vi "Controller.vi"(8 "error in":errorcluster) -> ()   [LabVIEW 2016, in "Vision Drive.lvlib"]
uses:
  Vision Drive.lvlib
  Target to Robot.ctl
  <vilib>/Analysis/coordinate.llb/Euler Rotation Order.ctl
  Constants/Private/Private Global.vi
  Private/Vision Target Global.vi
  Vision Server/Vision Server.lvclass
  Constants/Constants.lvlib
  <vilib>/Analysis/NI_AALPro.lvlib
  <vilib>/Analysis/coordinate.llb/3D Cartesian Coordinate Rotation (Euler) (Scalar).vi
panel:
  out "Pitch":dbl
  out "timestamp":u32
  out "Target Found?":bool
  out "Distance":dbl
  out "Angle":dbl
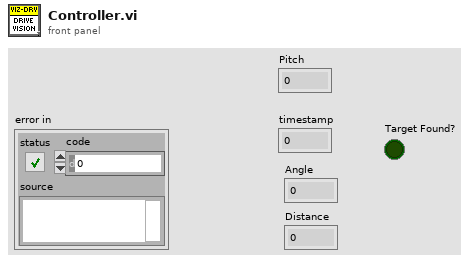
[diagram p1: front panel]
types:
  T1 = typedef "Constants.lvlib/Constants.ctl" = cluster{"Port Layout":cluster{"RightMotorInverted":bool, "LeftMotorInverted":bool, "Left Motors":T2, "Right Motors":T2, "Auton List":string[], "XBOX Port":T3, "Encoder L A":T4, "Encoder L B":T4, "Encoder R A":T4, "Encoder R B":T4, "L Encoder Inverse":bool, "R Encoder Inverse":bool, "Drive Distance per Count":dbl, "Gyro Bus":T5, "Fuel Roller 1":T2, "Front Roller":T2, "Gear Flipper":T2, "Climber 1":T2, "Fuel Roller Invert":bool, "Front Roller Invert":bool, "Gear Flipper Invert":bool, "Climber Invert":bool, "PCM":u8, "Fuel Roller 2":T2, "Gear Sensor":T6, "Gear Release Fwd":T7, "Gear Release Rvrs":T7, "Fuel Arm Fwd":T7, "Fuel Arm Rvrs":T7, "Shifter Fwrd":T7, "Shifter Rvrs":T7, "Climber 2":T2, "PDP":u8, "Shooter Front Channel":u8, "Shooter Rear Channel":u8, "Shooter Feed Channel":u8, "Camera Servo":T2, "Gear Servo":T2, "Gear Puncher Fwrd":T7, "Gear Puncher Rvrs":T7, "Shooter Inverse":bool, "Ring Light Switch":T4}, "Drive Constants":cluster{"Wheelbase In.":dbl, "Max Velocity (In/sec)":dbl, "Max Accel (In/sec^2)":dbl, "Max Jerk (In/sec^3)":dbl, "Path dt":dbl, "Path Sample Count":i32, "Deadband":dbl}, "Arm System":cluster{"Front Roller Gear Speed":dbl, "Front Roller Fuel Speed":dbl, "Gear Flipper Speed":dbl, "Fuel Roller Speed":dbl, "Gear Release Wait (ms)":i32, "Gear Sensor Threshold":dbl, "Flappy Open Angle":i32, "Flappy Close Angle":i32, "Ramp Rate (EGU/min)":dbl}, "Shooter":cluster{"Shooter Wheels":cluster{"P":dbl, "I":dbl, "D":dbl, "F":dbl, "IZone":dbl}, "Feeder":cluster{"P":dbl, "I":dbl, "D":dbl, "F":dbl, "IZone":dbl}, "Front Shooter RPM":dbl, "Rear Shooter RPM":dbl, "Agitator Speed":dbl, "Feeder Speed":dbl, "Shooter CPR":u32, "Feeder CPR":u32}, "Vision":cluster{"High Goal Height (in.)":dbl, "Low Goal Height (in.)":dbl, "Camera Height High (in.)":dbl, "Camera Height Low (in.)":dbl, "Servo Pitch Gear (deg)":dbl, "Camera Yaw (deg)":dbl, "Servo Gear":i32, "Servo Boiler":i32, "Servo Pitch Boiler (deg)":dbl}}
  T2 = typedef "FPGA_DIOPWMChannel.ctl" = enum8{"PWM 0", "PWM 1", "PWM 2", "PWM 3", "PWM 4", "PWM 5", "PWM 6", "PWM 7", "PWM 8", "PWM 9", "PWM MXP 0", "PWM MXP 1", "PWM MXP 2", "PWM MXP 3", "PWM MXP 4", "PWM MXP 5", "PWM MXP 6", "PWM MXP 7", "PWM MXP 8", "PWM MXP 9", "Invalid"}
  T3 = typedef "WPI_JoystickDeviceEnum.ctl" = enum16{"USB 0", "USB 1", "USB 2", "USB 3", "USB 4", "USB 5"}
  T4 = typedef "FPGA_DIOChannel.ctl" = enum8{"DIO 0", "DIO 1", "DIO 2", "DIO 3", "DIO 4", "DIO 5", "DIO 6", "DIO 7", "DIO 8", "DIO 9", "DIO MXP 0", "DIO MXP 1", "DIO MXP 2", "DIO MXP 3", "DIO MXP 4", "DIO MXP 5", "DIO MXP 6", "DIO MXP 7", "DIO MXP 8", "DIO MXP 9", "DIO MXP 10", "DIO MXP 11", "DIO MXP 12", "DIO MXP 13", "DIO MXP 14", "DIO MXP 15", "SPI Port CS1", "SPI Port CS2", "SPI Port CS3", "SPI Port MISO", "SPI Port MOSI", "Invalid"}
  T5 = typedef "spi_bus.ctl" = enum16{"SPI On-Board, CS0", "SPI On-Board, CS1", "SPI On-Board, CS2", "SPI On-Board, CS3", "SPI MXP", "Invalid"}
  T6 = typedef "FPGA_AIChannel.ctl" = enum8{"AI 0", "AI 1", "AI 2", "AI 3", "AI MXP 0", "AI MXP 1", "AI MXP 2", "AI MXP 3", "Invalid"}
  T7 = typedef "WPI_SolenoidChannel.ctl" = enum8{"Solenoid 0", "Solenoid 1", "Solenoid 2", "Solenoid 3", "Solenoid 4", "Solenoid 5", "Solenoid 6", "Solenoid 7", "Invalid"}
  T8 = cluster{"High Goal Height (in.)":dbl, "Low Goal Height (in.)":dbl, "Camera Height High (in.)":dbl, "Camera Height Low (in.)":dbl, "Servo Pitch Gear (deg)":dbl, "Camera Yaw (deg)":dbl, "Servo Gear":i32, "Servo Boiler":i32, "Servo Pitch Boiler (deg)":dbl}
  T9 = typedef "WPI_ServoDeviceRef.ctl" = cluster{"DeviceStatus":errorcluster, "PWM Channel":T2, "DeadBand":T10}
  T10 = typedef "WPI_PWMDeadband.ctl" = cluster{"Name":string, "maxPositivePwm":i32, "minPositivePwm":i32, "centerPwm":i32, "maxNegativePwm":i32, "minNegativePwm":i32, "angularRange":u16}
  T11 = typedef "Vision Server.lvclass/Target Listener Queue.ctl" = refnum<queue>
  T12 = cluster{"Vision":cluster{"High Goal Height (in.)":dbl, "Low Goal Height (in.)":dbl, "Camera Height High (in.)":dbl, "Camera Height Low (in.)":dbl, "Servo Pitch Gear (deg)":dbl, "Camera Yaw (deg)":dbl, "Servo Gear":i32, "Servo Boiler":i32, "Servo Pitch Boiler (deg)":dbl}, "ServoDeviceRef":T9, "Is Boiler?":bool, "Angle Thresh":u16}
  T13 = typedef "Vision Drive.lvlib/Target to Robot.ctl" = cluster{"Angle (deg)":dbl, "Distance (in)":dbl, "timestamp (ms)":u32, "Target Found":bool}
  T14 = typedef "Vision Server.lvclass/Target Vector.ctl" = cluster{"y":dbl, "z":dbl}
  T15 = typedef "NI_AALPro.lvlib/Euler Rotation Order.ctl" = u16
  T16 = typedef "Vision Server.lvclass/Sensor Message JSON.ctl" = cluster{"azimuth":dbl, "pitch":dbl, "roll":dbl}
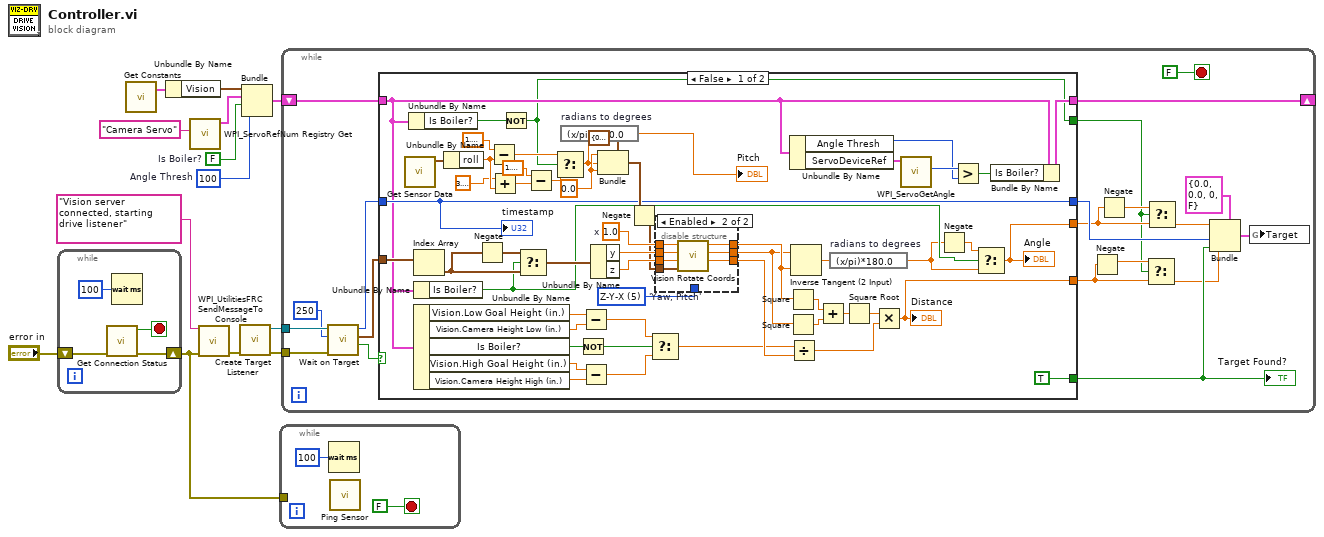
[diagram p0: block diagram]
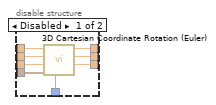
[diagram p2: hidden frame]
diagram:
  w2 = u16 100  # Angle Thresh
  w3 = FALSE  # Is Boiler?
  n1 = while {
    shift-right: [w14] -> w1
    shift-left: "error in" -> [w15]
    stop <- w17 stop-if-true
    n2 = call "Get Connection Status.vi"("error in"=w15) -> ("error out"=w14:errorcluster, "connected?"=w17:bool)  [unwired: 9 in]
    n3 = Wait (ms)(milliseconds to wait=u32 100) -> ()  [unwired: 1 out]
  }
  n4 = call "Get Constants.vi"() -> ("Constants"=w8:T1)  [unwired: 3 in]
  n5 = Unbundle By Name(w8) -> ("Vision"=w7:T8)
  n6 = call <vilib>:"WPI_ServoRefNum Registry Get.vi"("refnum name"="Camera Servo") -> ("ServoDeviceRef"=w5:T9)  [unwired: 9 in, 1 out]
  n7 = call <vilib>:"WPI_UtilitiesFRC SendMessageToConsole.vi"("Message"="Vision server connected, starting drive listener", "error in (no error)"=w1) -> ("error out"=w11:errorcluster)  [unwired: 13 in]
  n8 = call "Create Target Listener.vi"("error in"=w11) -> ("error out"=w10:errorcluster, "queue out"=w9:T11)  [unwired: 9 in]
  n9 = Bundle("Vision"=w7, "ServoDeviceRef"=w5, "Is Boiler?"=w3, "Angle Thresh"=w2) -> (w6:T12)  [unwired: 1 in]
  n10 = while {
    tunnel: w1 -> [_]
    stop <- FALSE stop-if-true
    n11 = Wait (ms)(milliseconds to wait=u32 100) -> ()  [unwired: 1 out]
    n12 = call "Ping Sensor.vi"() -> ()  [unwired: 11 in, 1 out]
  }
  n13 = while {
    tunnel: w10 -> [w37]
    tunnel: w9 -> [w38]
    shift-right: [w31] -> _
    shift-left: w6 -> [w32]
    stop <- FALSE stop-if-true
    # "Vision Update"
    n14 = call "Wait on Target.vi"("error in (no error)"=w37, "timeout in ms (-1)"=250, "queue in"=w38) -> ("timed out?"=w36:bool, "targets"=w33:T14[], "timestamp"=w34:u32)  [unwired: 5 in, 1 out]
    n15 = case shown="False" w36 {
      tunnel: w34 -> [w56 _]
      tunnel: w33 -> [w88 _]
      tunnel: [TRUE _] -> w28
      tunnel: w32 -> [w53 w110]
      tunnel: [w65 w110] -> w31
      tunnel: [w57 _] -> w24
      tunnel: [w66 _] -> w22
      tunnel: [w56 _] -> w27
      tunnel: [w40 _] -> w20
      frame False {
        w54 = 0.0 ("psi")
        w80 = T15 5 items=["X-Y-Z", "X-Z-Y", "Y-X-Z", "Y-Z-X", "Z-X-Y", "Z-Y-X", "X-Y-X", "X-Z-X", "Y-X-Y", "Y-Z-Y", "Z-X-Z", "Z-Y-Z"]  # 'Yaw, Pitch'
        w84 = 1.0  # x
        n16 = call "Get Sensor Data.vi"() -> ("Sensor"=w55:T16)  [unwired: 10 in, 1 out]
        n17 = Unbundle By Name(w53) -> ("Is Boiler?"=w41:bool)
        n18 = Index Array(array=w88) -> (element=w68:T14)  [unwired: 1 in]
        n19 = Unbundle By Name(w53) -> ("Is Boiler?"=w60:bool)
        n20 = Unbundle By Name(w53) -> ("Vision.Low Goal Height (in.)"=w77:dbl, "Vision.Camera Height Low (in.)"=w76:dbl, "Is Boiler?"=w78:bool, "Vision.High Goal Height (in.)"=w73:dbl, "Vision.Camera Height High (in.)"=w74:dbl)
        n21 = Unbundle By Name(w55) -> ("roll"=w49:dbl)
        n22 = Negate(x=w68) -> (-x=w69:T14)
        n23 = Subtract(x=1.5707963267948966, y=w49) -> (x-y=w46:dbl)
        n24 = Add(x=3.141592653589793, y=w49) -> (x+y=w44:dbl)
        n25 = Not(x=w41) -> (.not. x?=w40:bool)
        n26 = Select(t=w69, s=w60, f=w68) -> (s? t:f=w70:T14)
        n27 = Subtract(x=1.5707963267948966, y=w44) -> (x-y=w42:dbl)
        n28 = Select(t=w46, s=w40, f=w42) -> (s? t:f=w52:dbl)
        n29 = expression code="(x/pi)*180.0" "radians to degrees"(w52) -> (→"Pitch":dbl)
        n30 = Not(x=w78) -> (.not. x?=w50:bool)
        n31 = Subtract(x=w77, y=w76) -> (x-y=w75:dbl)
        n32 = Subtract(x=w73, y=w74) -> (x-y=w72:dbl)
        n33 = Unbundle By Name(w70) -> ("y"=w86:dbl, "z"=w85:dbl)
        n34 = Bundle(cluster=cluster{"phi":dbl, "theta":dbl, "psi":dbl} {"phi"=0.0, "theta"=0.0, "psi"=0.0} ("Euler Angles"), "phi"=w54, "theta"=w52, "psi"=w54) -> (w71:cluster{"phi":dbl, "theta":dbl, "psi":dbl})
        n35 = Negate(x=w71) -> (-x=w45:cluster{"phi":dbl, "theta":dbl, "psi":dbl})
        n36 = Select(t=w75, s=w50, f=w72) -> (s? t:f=w67:dbl)
        n37 = disable-structure shown="Enabled" {
          disable-tunnel: w86 -> [w102 w107]
          disable-tunnel: w85 -> [w101 w108]
          disable-tunnel: w84 -> [w100 w106]
          disable-tunnel: [w99 w105] -> w83
          disable-tunnel: [w98 w104] -> w82
          disable-tunnel: [w97 w103] -> w81
          disable-tunnel: w80 -> [w96 _]
          disable-tunnel: w45 -> [w95 w109]
          frame Disabled {
            n38 = call-poly <vilib>:"3D Cartesian Coordinate Rotation (Euler).vi"("rotation order"=w96, "Euler Angles"=w95, "z"=w101, "y"=w102, "x"=w100) -> ("z out"=w97:dbl, "y out"=w98:dbl, "x out"=w99:dbl)  [unwired: 3 in, 1 out]
          }
          frame Enabled {
            n39 = call "Vision Rotate Coords.vi"("output cluster"=w109, "z"=w108, "y"=w107, "x"=w106) -> ("zr"=w103:dbl, "yr"=w104:dbl, "xr"=w105:dbl)  [unwired: 5 in]
          }
        }
        n40 = Square(x=w83) -> (x^2=w93:dbl)
        n41 = Square(x=w82) -> (x^2=w92:dbl)
        n42 = Divide(x=w67, y=w81) -> (x/y=w89:dbl)
        n43 = Unbundle By Name(w53) -> ("Angle Thresh"=w62:u16, "ServoDeviceRef"=w64:T9)
        n44 = Inverse Tangent (2 Input)(1:w83, 2:w82) -> (0:w94:dbl)
        n45 = Add(x=w93, y=w92) -> (x+y=w91:dbl)
        n46 = expression code="(x/pi)*180.0" "radians to degrees"(w94) -> (w58:dbl)
        n47 = Square Root(x=w91) -> (sqrt(x)=w90:dbl)
        n48 = Multiply(x=w90, y=w89) -> (x*y=w66:dbl)
        "Distance" <- w66
        n49 = call <vilib>:"WPI_ServoGetAngle.vi"("ServoDeviceRef"=w64) -> ("Angle"=w63:u16)  [unwired: 7 in, 2 out]
        n50 = Negate(x=w58) -> (-x=w59:dbl)
        n51 = Greater?(x=w63, y=w62) -> (0:w61:bool)
        n52 = Select(t=w59, s=w60, f=w58) -> (s? t:f=w57:dbl)
        "Angle" <- w57
        n53 = Bundle By Name(cluster=w53, "Is Boiler?"=w61) -> (w65:T12)
        "timestamp" <- w56
      }
      frame True {
      }
    }
    "Target Found?" <- w28
    n54 = Negate(x=w22) -> (-x=w21:dbl)
    n55 = Negate(x=w24) -> (-x=w25:dbl)
    n56 = Select(t=w21, s=w20, f=w22) -> (s? t:f=w23:dbl)
    n57 = Select(t=w25, s=w20, f=w24) -> (s? t:f=w26:dbl)
    n58 = Bundle(cluster=T13 {"Angle (deg)"=0.0, "Distance (in)"=0.0, "timestamp (ms)"=0, "Target Found"=FALSE}, "Angle (deg)"=w26, "Distance (in)"=w23, "timestamp (ms)"=w27, "Target Found"=w28) -> (w29:T13)
    n59 = global write "Vision Target Global.vi" "Target"(w29) -> ()
  }
